vi "Log Init.vi"(6 "Configuration":T2={"Accelerometer Bias"={"X (m/s)"=0.0, "Y (m/s)"=0.0, "Z (m/s)"=0.0}, "Gyroscope Bias"={"X (m/s)"=0.0, "Y (m/s)"=0.0, "Z (m/s)"=0.0}, "Steering Motor Gear Ratio"=611.0, "Steering Pully Gear Ratio"=1.0, "Steering Encoder CPR"=500.0, "Steering Motor Max RPM"=4000.0, "Wheelbase (m)"=1.12, "Fork Angle (rad)"=1.3, "Balancing Controller"={"Kp (/s)"=0.0, "Kd (1)"=0.0}, "Max Allowed Steering Angle (rad)"=0.7, "Task Periods"={"Emergency Stop (us)"=0, "IMU (us)"=0, "Steering Motor Encoder (us)"=0, "State Estimator (us)"=0, "Balancing Controller (us)"=0, "GNSS (us)"=0, "Logging (us)"=0, "Drive Motor (us)"=0, "Visualization (us)"=50000}, "Drive Motor Gear Ratio"=0.7, "lr"=0.0, "lf"=0.0, "lambda"=0.0, "k1"=0.0, "k2"=0.0, "e1_max"=0.0, "Ad_tmin"=0.0, "Bd_tmin"=0.0, "C_tmin"=0.0, "D_tmin"=0.0, "Wheel radius"=0.311, "Ad_tmax"=0.95971, "Bd_tmax"=0.01, "C_tmax"=2.20588, "D_tmax"=0.0, "Vmin"=2.20588, "Vmax"=0.0}, 8 "Matrices":T1, 9 "Trajectory":dbl[][](array[numeric]), 11 "Error In":errorcluster) -> (2 "Log Handle":T3, 3 "Error Out":errorcluster)   [LabVIEW 2021]
uses:
  Log Handle.ctl
  Configuration/Configuration.ctl
  <vilib>/Analysis/Matrix/Datatypes/RealMatrix.ctl
  <vilib>/Analysis/Matrix/NI_Matrix.lvlib
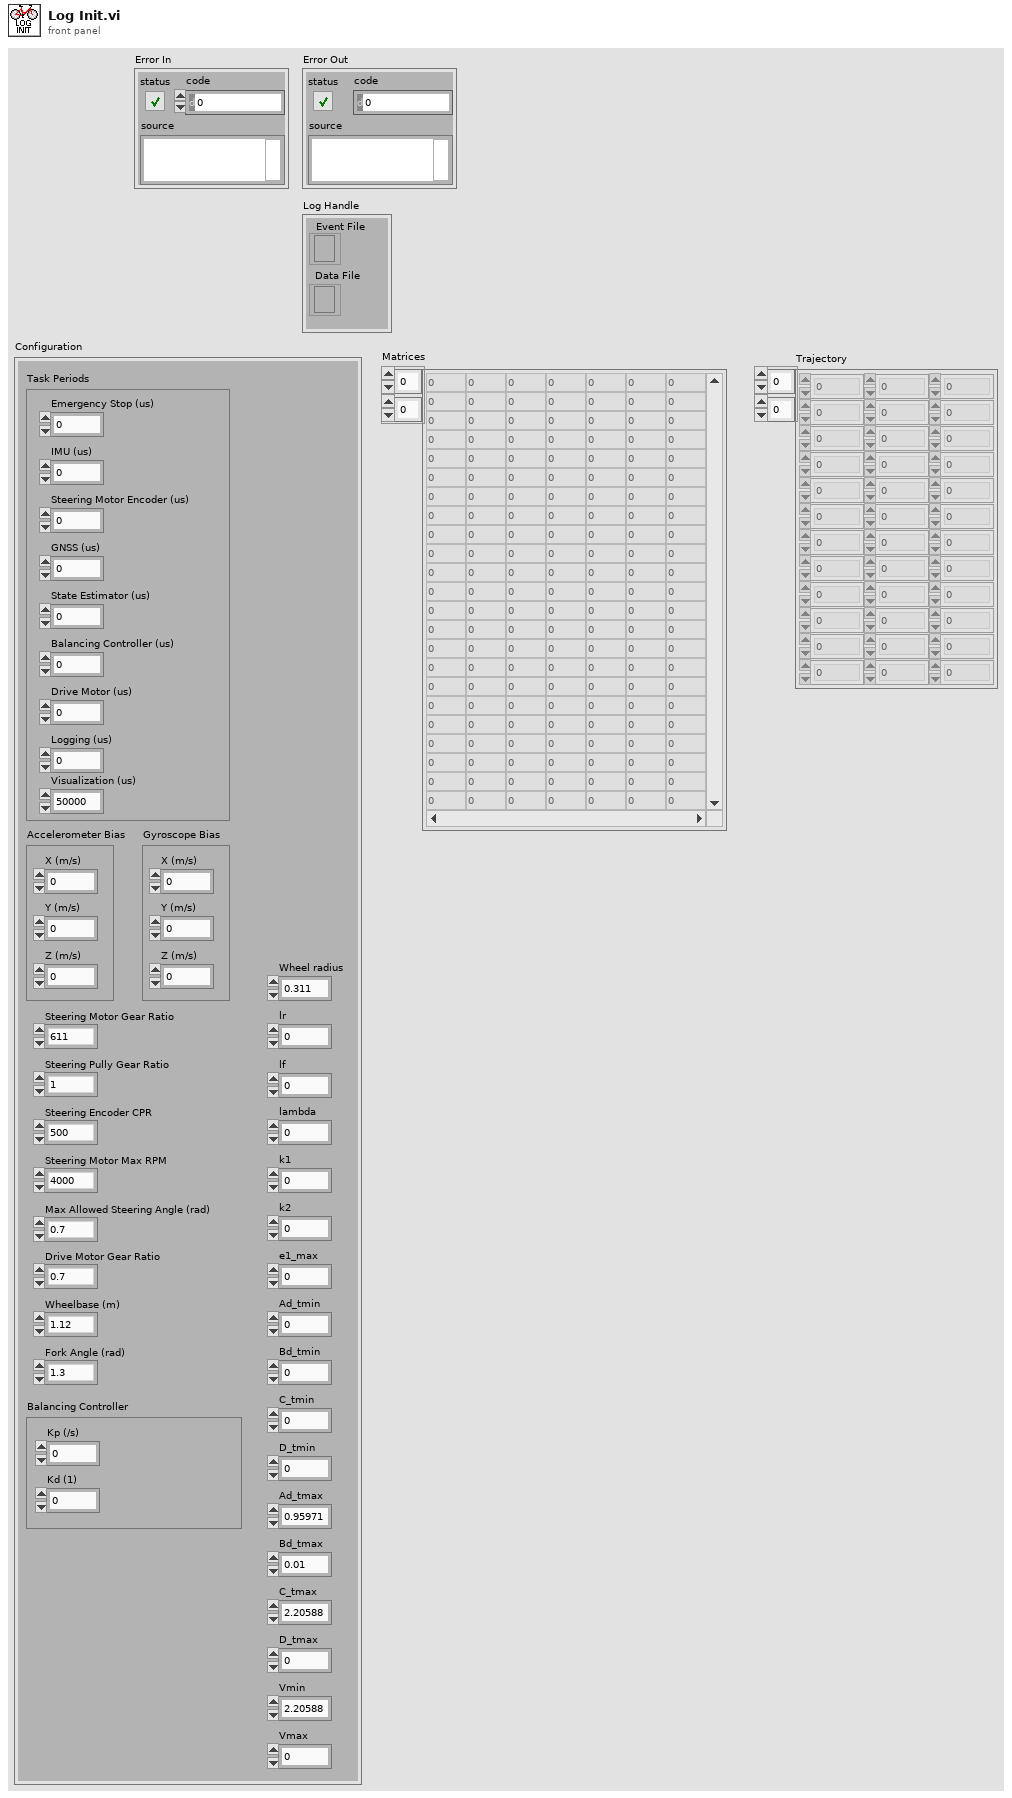
[diagram p1: front panel]
types:
  T1 = typedef "NI_Matrix.lvlib/RealMatrix.ctl" = dbl[][]
  T2 = typedef "Configuration.ctl" = cluster{"Accelerometer Bias":cluster{"X (m/s)":dbl, "Y (m/s)":dbl, "Z (m/s)":dbl}, "Gyroscope Bias":cluster{"X (m/s)":dbl, "Y (m/s)":dbl, "Z (m/s)":dbl}, "Steering Motor Gear Ratio":dbl, "Steering Pully Gear Ratio":dbl, "Steering Encoder CPR":dbl, "Steering Motor Max RPM":dbl, "Wheelbase (m)":dbl, "Fork Angle (rad)":dbl, "Balancing Controller":cluster{"Kp (/s)":dbl, "Kd (1)":dbl}, "Max Allowed Steering Angle (rad)":dbl, "Task Periods":cluster{"Emergency Stop (us)":i64, "IMU (us)":i64, "Steering Motor Encoder (us)":i64, "State Estimator (us)":i64, "Balancing Controller (us)":i64, "GNSS (us)":i64, "Logging (us)":i64, "Drive Motor (us)":i64, "Visualization (us)":i64}, "Drive Motor Gear Ratio":dbl, "lr":dbl, "lf":dbl, "lambda":dbl, "k1":dbl, "k2":dbl, "e1_max":dbl, "Ad_tmin":dbl, "Bd_tmin":dbl, "C_tmin":dbl, "D_tmin":dbl, "Wheel radius":dbl, "Ad_tmax":dbl, "Bd_tmax":dbl, "C_tmax":dbl, "D_tmax":dbl, "Vmin":dbl, "Vmax":dbl}
  T3 = typedef "Log Handle.ctl" = cluster{"Data File":refnum<file>, "Event File":refnum<file>}
  T4 = enum16{"open", "replace", "create", "open or create", "replace or create", "replace or create with confirmation"}
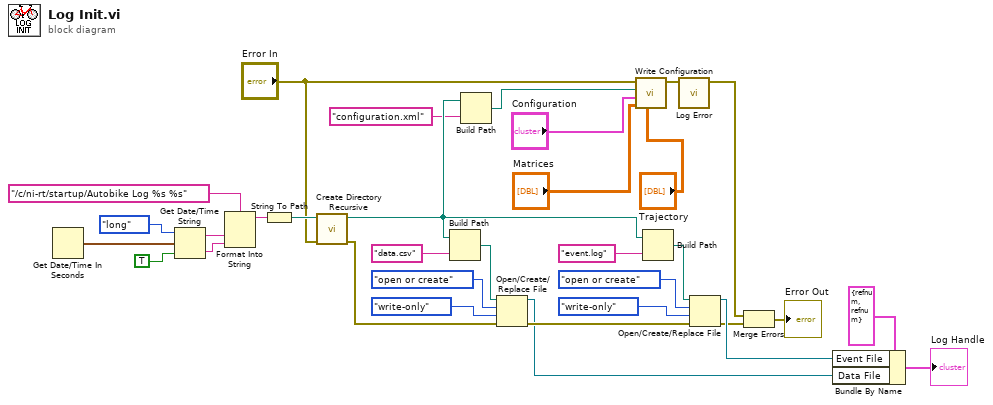
[diagram p0: block diagram]
diagram:
  n1 = Get Date/Time In Seconds() -> (seconds since 1Jan1904=w33:timestamp)
  n2 = Get Date/Time String(date format (0)=enum16{"short", "long", "abbreviated"}."long", seconds (now)=w33, want seconds? (F)=TRUE) -> (date string=w29:string, time string=w28:string)
  n3 = Format Into String(format string="/c/ni-rt/startup/Autobike Log %s %s", w29, w28) -> (resulting string=w25:string)  [unwired: 2 in, 1 out]
  n4 = String To Path(string=w25) -> (path=w22:path)
  n5 = call <vilib>:"Create Directory Recursive.vi"("error in (no error)"="Error In", "directory"=w22) -> ("error out"=w21:errorcluster, "directory copy"=w8:path)  [unwired: 3 in, 1 out]
  n6 = Build Path(base path=w8, name or relative path="data.csv") -> (appended path=w24:path)
  n7 = Build Path(base path=w8, name or relative path="configuration.xml") -> (appended path=w6:path)
  n8 = Open/Create/Replace File(file path (use dialog)=w24, error in=w21, operation (0:open)=T4."open or create", access (0:read/write)=enum16{"read/write", "read-only", "write-only"}."write-only") -> (refnum out=w13:refnum<file>, error out=w14:errorcluster)  [unwired: 2 in, 1 out]
  n9 = call "Write Configuration.vi"("Array"="Trajectory", "Real Matrix"="Matrices", "Configuration"="Configuration", "XML File Path conf"=w6, "Error In"="Error In") -> ("Error Out"=w5:errorcluster)  [unwired: 6 in]
  n10 = Build Path(base path=w8, name or relative path="event.log") -> (appended path=w18:path)
  n11 = call "Log Error.vi"("Error In"=w5) -> ("Error Out"=w4:errorcluster)  [unwired: 10 in]
  n12 = Open/Create/Replace File(file path (use dialog)=w18, error in=w14, operation (0:open)=T4."open or create", access (0:read/write)=enum16{"read/write", "read-only", "write-only"}."write-only") -> (refnum out=w12:refnum<file>, error out=w10:errorcluster)  [unwired: 2 in, 1 out]
  n13 = Merge Errors(w4, w10) -> (→"Error Out":errorcluster)
  n14 = Bundle By Name(cluster=T3 {"Data File"=refnum, "Event File"=refnum} ("Log Handle"), "Event File"=w12, "Data File"=w13) -> (→"Log Handle":T3)
